vi "Receive Time Info.vi"(8 "error in":errorcluster, 9 "Elapsed Time":dbl, 10 "Elapsed?":bool, 11 "Platform in":refnum<class "Platform.lvclass">) -> (0 "error out":errorcluster, 3 "Platform out":refnum<class "Platform.lvclass">)   [LabVIEW 2019, in "Platform.lvlib" / "Platform.lvclass"]
uses:
  Platform.lvclass
  C:/Program Files (x86)/National Instruments/LabVIEW 2019/vi.lib/ActorFramework/Actor/Actor.lvclass
  <vilib>/ActorFramework/Actor/Actor.lvclass/Actor.ctl
  <vilib>/ActorFramework/Message Enqueuer/Message Enqueuer.lvclass/Message Enqueuer.ctl
  Platform.lvclass/Platform.ctl
  Timer/Timer Messages/Start Timer Msg/Start Timer Msg.lvclass/Start Timer Msg.ctl
  Platform Messages/Run Msg/PF Commands Msg.lvclass/PF Commands Msg.ctl
  Platform Messages/Get Status Msg/Get Status Msg.lvclass/Get Status Msg.ctl
  <vilib>/ActorFramework/Message Enqueuer/Init from Existing Queue.vi
  <vilib>/ActorFramework/Message Enqueuer/Enqueue.vi
  Timer/Timer Messages/Start Timer Msg/Start Timer Msg.lvclass
  C:/Program Files (x86)/National Instruments/LabVIEW 2019/vi.lib/ActorFramework/Message/Message.lvclass
  Platform Messages/Run Msg/PF Commands Msg.lvclass
  Platform Messages/Get Status Msg/Get Status Msg.lvclass
  <vilib>/ActorFramework/Message Priority Queue/Priority Enqueue.vi
  <vilib>/ActorFramework/Message Enqueuer/Message Enqueuer.lvclass
  <vilib>/ActorFramework/Actor/Actor.lvclass
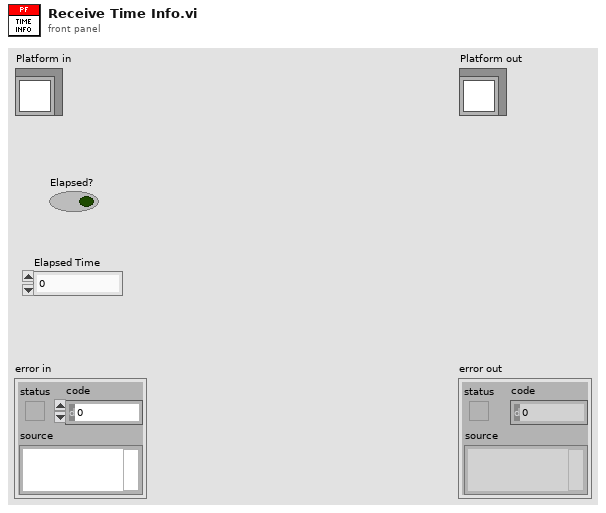
[diagram p1: front panel]
types:
  T1 = enum8{"Enabled", "Disabled", "Disabled and Grayed Out"}
  T2 = cluster{"Duration":i32, "Value":u32, "Name":string}[]
  T3 = cluster{"Duration":i32, "Value":u32, "Name":string}
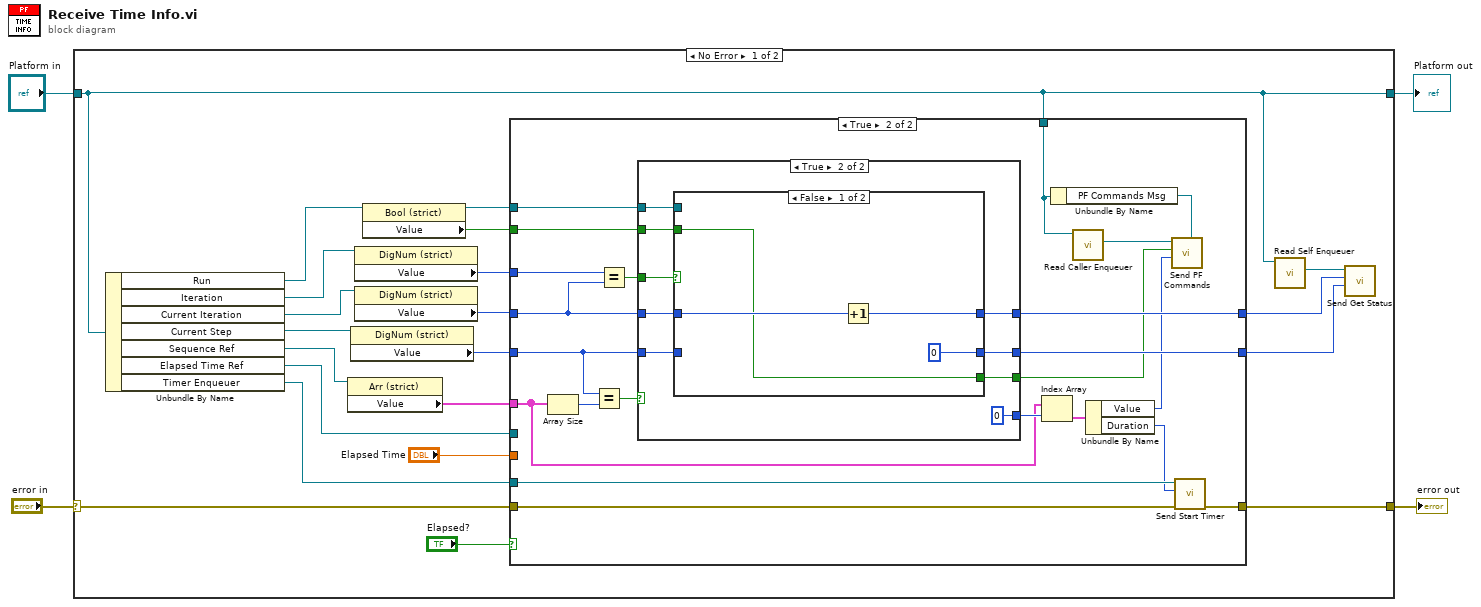
[diagram p0: block diagram]
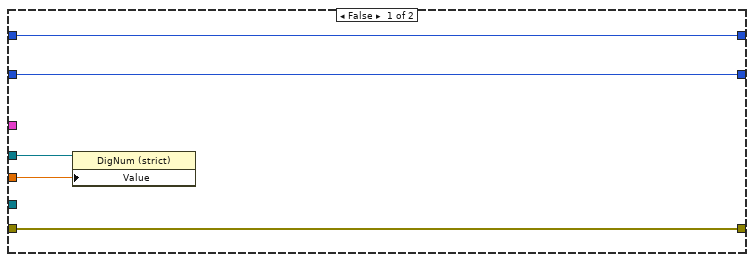
[diagram p2: hidden frame]
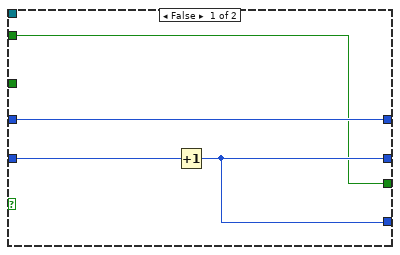
[diagram p3: hidden frame]
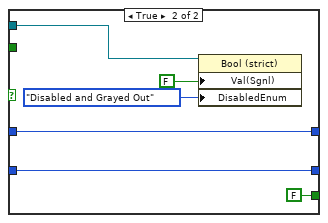
[diagram p4: hidden frame]
diagram:
  n1 = case shown="No Error" "error in" {
    selector: "error in" -> [w20 w77]
    tunnel: [w9 w77] -> w3
    tunnel: [w5 w76] -> w1
    tunnel: "Platform in" -> [w5 w76]
    frame No Error {
      n2 = Unbundle By Name(w5) -> ("Run"=w8:refnum<vi>, "Iteration"=w15:refnum<vi>, "Current Iteration"=w17:refnum<vi>, "Current Step"=w19:refnum<vi>, "Sequence Ref"=w25:refnum<vi>, "Elapsed Time Ref"=w10:refnum<vi>, "Timer Enqueuer"=w21:refnum<class "Message Enqueuer.lvclass">)
      n3 = property class="Arr (strict)"(reference=w25) -> ("Value"=w24:T2)  [unwired: 1 in, 2 out]
      n4 = property class="DigNum (strict)"(reference=w19) -> ("Value"=w18:i32)  [unwired: 1 in, 2 out]
      n5 = property class="DigNum (strict)"(reference=w15) -> ("Value"=w14:i32)  [unwired: 1 in, 2 out]
      n6 = property class="DigNum (strict)"(reference=w17) -> ("Value"=w16:i32)  [unwired: 1 in, 2 out]
      n7 = property class="Bool (strict)"(reference=w8) -> (reference out=w6:refnum<vi>, "Value"=w7:bool)  [unwired: 1 in, 1 out]
      n8 = case shown="True" "Elapsed?" {
        tunnel: [w26 w52] -> w11
        tunnel: w18 -> [w26 w50]
        tunnel: w16 -> [w30 w45]
        tunnel: w14 -> [_ w46]
        tunnel: w20 -> [w29 w43]
        tunnel: [w29 w42] -> w9
        tunnel: [w30 w47] -> w12
        tunnel: w24 -> [_ w38]
        tunnel: w10 -> [w28 _]
        tunnel: "Elapsed Time" -> [w27 _]
        tunnel: w21 -> [_ w44]
        tunnel: w7 -> [_ w37]
        tunnel: w6 -> [_ w36]
        tunnel: w5 -> [_ w33]
        frame False {
          n9 = property class="DigNum (strict)"(reference=w28, "Value"=w27) -> ()  [unwired: 1 in, 2 out]
        }
        frame True {
          n10 = Array Size(array=w38) -> (size(s)=w51:i32)
          n11 = Equal?(x=w50, y=w51) -> (x = y?=w49:bool)
          n12 = Equal?(x=w46, y=w45) -> (x = y?=w48:bool)
          n13 = case shown="True" w49 {
            tunnel: w48 -> [_ w65]
            tunnel: w45 -> [w56 w64]
            tunnel: [w56 w63] -> w47
            tunnel: [w54 0] -> w39
            tunnel: w50 -> [w55 w61]
            tunnel: [w54 w62] -> w52
            tunnel: w37 -> [w53 w59]
            tunnel: [w53 w58] -> w31
            tunnel: w36 -> [_ w57]
            frame False {
              n14 = Increment(x=w55) -> (x+1=w54:i32)
            }
            frame True {
              n15 = case shown="False" w65 {
                tunnel: w64 -> [w69 w74]
                tunnel: [w68 w74] -> w63
                tunnel: [0 ("index") w73] -> w62
                tunnel: w61 -> [_ w73]
                tunnel: w59 -> [w66 _]
                tunnel: [w66 FALSE] -> w58
                tunnel: w57 -> [_ w70]
                frame False {
                  n16 = Increment(x=w69) -> (x+1=w68:i32)
                }
                frame True {
                  n17 = property class="Bool (strict)"(reference=w70, "Val(Sgnl)"=FALSE ("Run"), "DisabledEnum"=T1."Disabled and Grayed Out" ("Disabled")) -> ()  [unwired: 1 in, 2 out]
                }
              }
            }
          }
          n18 = Index Array(array=w38, index=w39) -> (element=w41:T3)
          n19 = Unbundle By Name(w33) -> ("PF Commands Msg"=w35:refnum<class "PF Commands Msg.lvclass">)
          n20 = call <vilib>:"Read Caller Enqueuer.vi"("Actor"=w33) -> ("Caller Enqueuer"=w34:refnum<class "Message Enqueuer.lvclass">)  [unwired: 10 in]
          n21 = Unbundle By Name(w41) -> ("Value"=w32:u32, "Duration"=w40:i32)
          n22 = call "Send PF Commands.vi"("Message Type"=w35, "Setpoint"=w32, "Run"=w31, "Message Enqueuer"=w34) -> ()  [unwired: 6 in, 2 out]
          n23 = call "Send Start Timer.vi"("error in (no error)"=w43, "Time Target (s)"=w40, "Message Enqueuer"=w44) -> ("error out"=w42:errorcluster)  [unwired: 7 in, 1 out]
        }
      }
      n24 = call <vilib>:"Read Self Enqueuer.vi"("Actor"=w5) -> ("Self Enqueuer"=w13:refnum<class "Message Enqueuer.lvclass">)  [unwired: 10 in]
      n25 = call "Send Get Status.vi"("Current Step"=w11, "Current Iteration"=w12, "Message Enqueuer"=w13) -> ()  [unwired: 7 in, 2 out]
    }
    frame Error {
    }
  }
  "error out" <- w3
  "Platform out" <- w1
